vi "worksheet filter column2.vi"(6 "and_or":u8, 7 "rule2":u32, 8 "error in (no error)":errorcluster, 9 "rule1":u32, 10 "col":u16, 11 "worksheet":u32) -> (0 "error out":errorcluster, 3 "function return":u32(ring))   [LabVIEW 8.6]
doc: "lxw_error worksheet_filter_column2(lxw_worksheet worksheet, lxw_col_t col, unsigned long rule1, unsigned long rule2, uint8_t and_or);"
uses:
  pending_lvxlsxwriter/xlsxwriter.dll
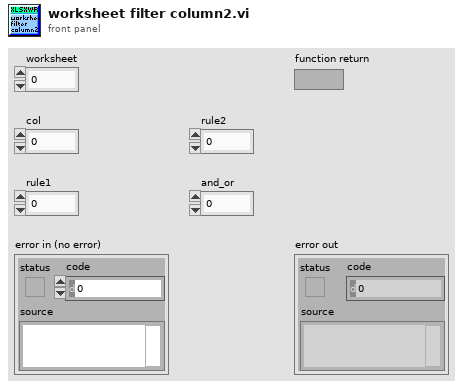
[diagram p1: front panel]
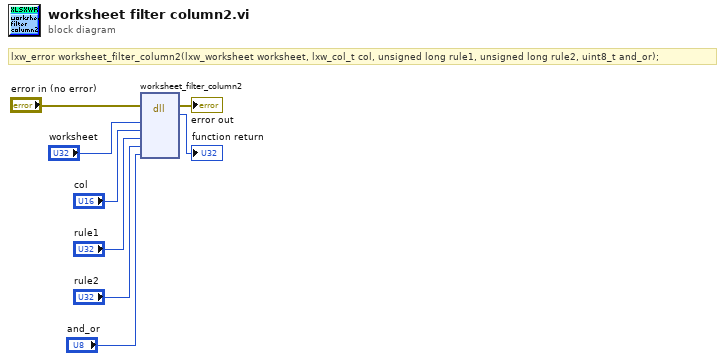
[diagram p0: block diagram]
diagram:
  # "lxw_error worksheet_filter_column2(lxw_worksheet worksheet, lxw_col_t col, unsigned long rule1, unsigned long rule2, uint8_t and_or);"
  n1 = dll-call lib="C:/Users/WDAGUtilityAccount/Desktop/pending_lvxlsxwriter/xlsxwriter.*" fn="worksheet_filter_column2"(error in="error in (no error)", "worksheet"="worksheet", "col"="col", "rule1"="rule1", "rule2"="rule2", "and_or"="and_or") -> (error out=→"error out":errorcluster, →"function return":u32)  [unwired: 7 in, 1 out]
